vi "SetInitialPlayerPositions_Fixed.vi"(8 "error in (no error)":errorcluster, 9 "Player2Position":T1, 10 "Player1Position":T1, 11 "Board in":refnum<class "Board.lvclass">) -> (0 "error out":errorcluster, 3 "Board out":refnum<class "Board.lvclass">)   [LabVIEW 2015, in "TronviewGame.lvlib" / "GameBuilder.lvclass"]
uses:
  GameBuilder.lvclass
  Board/Board.lvclass
  Board/Position.ctl
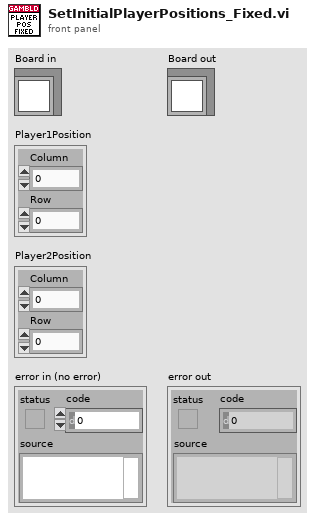
[diagram p1: front panel]
types:
  T1 = typedef "TronviewGame.lvlib/Board.lvclass/Position.ctl" = cluster{"Column":i32, "Row":i32}
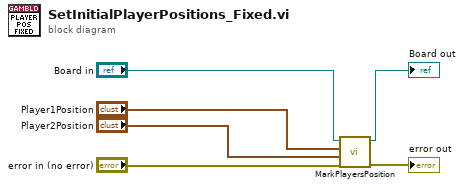
[diagram p0: block diagram]
diagram:
  n1 = call "MarkPlayersPosition.vi"("error in (no error)"="error in (no error)", "Player2NewPosition"="Player2Position", "Player1NewPosition"="Player1Position", "Board in"="Board in") -> ("error out"=→"error out":errorcluster, "Board out"=→"Board out":refnum<class "Board.lvclass">)  [unwired: 4 in, 2 out]
